vi "1.0-Hindbrain Global.vi"() -> ()   [LabVIEW 2010]
uses:
  2-Low Neurons/2.0-Hindbrain Startup State.ctl
  2-Low Neurons/2.1-Act Command Typedef.ctl
  2-Low Neurons/2.1 PID Gains Typedef.ctl
  2-Low Neurons/2.3-What Sensor Typedef.ctl
  2-Low Neurons/Data Latch.ctl
  2-Low Neurons/2.4-How Sensor Typedef.ctl
  2-Low Neurons/2.3.6-Decode State.ctl
  2-Low Neurons/2.7-Sense Queries Typedef.ctl
panel:
  out "Stop Loops":bool
  in  "Tab, for convenience":T1(tab)
  in  "2.1.3 Lidar Error D":fxp<+/-,18,1>
  in  "2.1.3 Lidar Error I":fxp<+/-,64,46>
  in  "2.1.3 Lidar Error":fxp<+/-,18,1>
  in  "2.1.2 Steering Error D":fxp<+/-,18,1>
  in  "2.1.2 Steering Error I":fxp<+/-,64,46>
  in  "2.1.2 Steering Error":fxp<+/-,18,1>
  in  "2.1.1 Drive Error D":fxp<+/-,18,1>
  in  "2.1.1 Drive Error I":fxp<+/-,64,46>
  in  "2.1.1 Drive Error":fxp<+/-,18,1>
  in  "2.1  Drive PID Output":fxp<+/-,20,5>
  in  "2.1  Lidar PID Output":fxp<+/-,20,5>
  in  "2.1  Steering PID Output":fxp<+/-,20,5>
  in  "2.1  Lidar Control Voltage":fxp<+/-,20,5>
  in  "2.1  Steering Control Voltage":fxp<+/-,20,5>
  in  "2.1 Drive Control Voltage":fxp<+/-,20,5>
  in  "2.1 Act Command":T2={"Inhibit All Motors"=FALSE, "2.1 Direct Override"=FALSE, "Drive Speed Integer Setpoint"=0, "Steering Integer Setpoint"=0, "Lidar Position Integer Setpoint"=0, "Drive Direct"=0.0, "Steer Direct"=0.0, "Lidar Direct "=0.0, "2.1.3 Drive PID Gains"={"P Gain"=0.25, "I Gain"=0.25, "D Gain"=0.25, "P Gain - Exp"=2, "I Gain - Exp"=2, "D Gain - Exp"=2}, "2.1.3 Steering PID Gains"={"P Gain"=0.25, "I Gain"=0.25, "D Gain"=0.25, "P Gain - Exp"=2, "I Gain - Exp"=2, "D Gain - Exp"=2}, "2.1.3 Lidar PID Gains"={"P Gain"=0.25, "I Gain"=0.25, "D Gain"=0.25, "P Gain - Exp"=2, "I Gain - Exp"=2, "D Gain - Exp"=2}, "2.5.5 A"=0.0, "2.5.6 B"=0.0, "Drive Limit"=0.0} {"2.1.3 Lidar PID Gains"."P Gain" format="%.8f"; "2.1.3 Lidar PID Gains"."I Gain" format="%.8f"; "2.1.3 Lidar PID Gains"."D Gain" format="%.8f"; "2.1.3 Drive PID Gains"."P Gain" format="%.8f"; "2.1.3 Drive PID Gains"."I Gain" format="%.8f"; "2.1.3 Drive PID Gains"."D Gain" format="%.8f"; "2.1.3 Steering PID Gains"."P Gain" format="%.8f"; "2.1.3 Steering PID Gains"."I Gain" format="%.8f"; "2.1.3 Steering PID Gains"."D Gain" format="%.8f"}
  out "2.2.4-VectorNav Query":bool
  out "2.2.4 Read TimedOut?":bool
  out "2.2.3 Write TimedOut?":bool
  out "2.2.2 VectorNav ReceivedByte":u8
  in  "2.2.2 VectorNav SendByte":u8
  in  "2.2.1 VectorNavCommand":u8[](array[numeric])=[36, 86, 78, 82, 82, 71, 44, 48, 46, 52, 55, 66]
  in  "2.2.1Send":bool
  in  "2.2.1 VectorNav Yaw":i16
  in  "2.2 Where am I? Sensor":T4
  in  "2.3 What is Around Me? Sensor":T5={"FPGA Raw Datalatch"=enum."Idle", "Drivable Path Integers"=[0, 0, 0, 0, 0, 0, 0, 0, 0, 0, 0, 0, 0, 0, 0, 0]}
  out "2.3.6-Decode State":T7
  out "2.3.3-Scan":u8
  out "2.3.7-Paths":u16[](array[numeric])
  out "2.3.4-X":i16
  out "2.3.5-Y":i16
  out "2.3.8-DMA Timeout":bool
  in  "2.4.5 FPGA LED Heart Beat Duty":u8
  in  "2.4.2.3 Reverse?":bool
  in  "2.4.4.2 Lidar V":fxp<+/-,10,8>
  in  "2.4.3.2 Lidar Mot V":fxp<+/-,10,8>
  in  "2.4.1.2 Steer V":fxp<+/-,10,8>
  in  "2.4.2.2 Drive V":fxp<+/-,10,8>
  in  "2.4.4.1 Lidar Pos":i32
  in  "2.4.3.1 Lidar Mot Pos":i32
  in  "2.4.2.1 Drive Pos":i32
  in  "2.4.1.1 Steer Pos":i32
  in  "2.4 How Am I? Sensor":T8
  in  "2.5.7 A*B":fxp<+/-,18,1>
  out "2.5.4-Timeouts by Identifier":bool[](array[boolean])
  in  "2.5.1-Write Index":u32
  out "2.7 Sense Queries":T9
  in  "Enum":T10=enum."Running"
  # "2.5.2-MultServ Out"
  # "2.5.3-MultServ In"
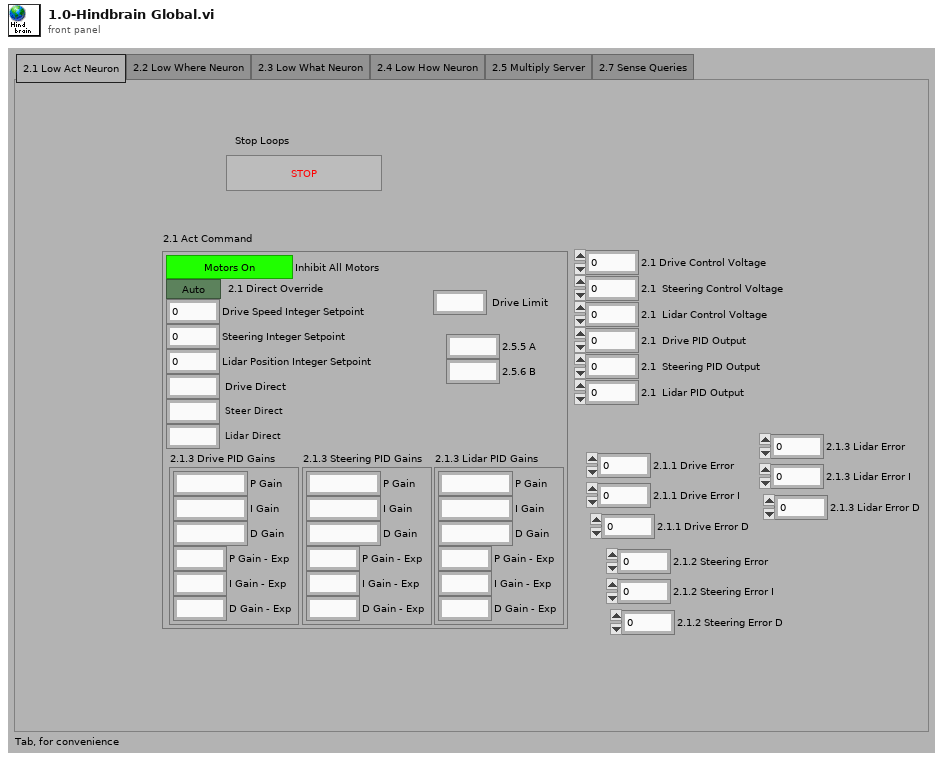
[diagram p1: front panel]
types:
  T1 = enum32{"2.1 Low Act Neuron", "2.2 Low Where Neuron", "2.3 Low What Neuron", "2.4 Low How Neuron", "2.5 Multiply Server", "2.7 Sense Queries"}
  T2 = typedef "2.1-Act Command Typedef.ctl" = cluster{"Inhibit All Motors":bool, "2.1 Direct Override":bool, "Drive Speed Integer Setpoint":i32, "Steering Integer Setpoint":i32, "Lidar Position Integer Setpoint":i32, "Drive Direct":fxp<+/-,20,5>, "Steer Direct":fxp<+/-,20,5>, "Lidar Direct ":fxp<+/-,20,5>, "2.1.3 Drive PID Gains":T3, "2.1.3 Steering PID Gains":T3, "2.1.3 Lidar PID Gains":T3, "2.5.5 A":fxp<+/-,18,1>, "2.5.6 B":fxp<+/-,18,1>, "Drive Limit":fxp<+/-,20,5>}
  T3 = typedef "2.1 PID Gains Typedef.ctl" = cluster{"P Gain":fxp<+/-,18,1>, "I Gain":fxp<+/-,18,1>, "D Gain":fxp<+/-,18,1>, "P Gain - Exp":i8, "I Gain - Exp":i8, "D Gain - Exp":i8}
  T4 = cluster{"INS X":i16, "INS Y":i16, "INS Z":i16, "INS Yaw":i16, "INS Raw":i8}
  T5 = typedef "2.3-What Sensor Typedef.ctl" = cluster{"FPGA Raw Datalatch":T6, "Drivable Path Integers":u16[]}
  T6 = typedef "Data Latch.ctl" = enum8{"Idle", "Sending", "Sent", "Receiving", "Received"}
  T7 = typedef "2.3.6-Decode State.ctl" = enum16{"wait for message start '['", "wait for point start '(' ", "record x value", "record y value", "scan complete"}
  T8 = typedef "2.4-How Sensor Typedef.ctl" = cluster{"Motor Speed Integer":i32, "Drive Position Integer":i32, "Lidar Position Integer":i32, "Lidar Motor Position Integer":i32, "Steering Position Integer":i32, "Battery Voltage Fxp":fxp<+/-,16,5>, "Drive Encoder Cable Check":bool, "Lidar Drive Encoder Cable Check":bool, "Steer Encoder Cable Check":bool, "Lidar Pos Encoder Cable Check":bool, "Mod Buttons & Blinky Cable Check":bool, "Lidar Data Cable Check":bool, "Drive Motor Cable Check":bool, "Vector Nav Cable Check":bool, "Lidar Drive Cable Check":bool, "Steer Drive Cable Check":bool, "Reverse?":bool, "2.1  Steering Control Voltage":fxp<+/-,20,5>, "2.1 Drive Control Voltage":fxp<+/-,20,5>, "2.1  Lidar Control Voltage":fxp<+/-,20,5>, "2.5.7 A*B":fxp<+/-,18,1>, "2.1  Steering PID Output":fxp<+/-,20,5>, "2.1 Drive PID Output":fxp<+/-,20,5>, "2.1  Lidar PID Output":fxp<+/-,20,5>, "2.1.1 Drive Error":fxp<+/-,18,1>, "2.1.1 Drive Error I":fxp<+/-,64,46>, "2.1.1 Drive Error D":fxp<+/-,18,1>, "2.1.2 Steering Error":fxp<+/-,18,1>, "2.1.2 Steering Error I":fxp<+/-,64,46>, "2.1.2 Steering Error D":fxp<+/-,18,1>, "2.1.3 Lidar Error":fxp<+/-,18,1>, "2.1.3 Lidar Error I":fxp<+/-,64,46>, "2.1.3 Lidar Error D":fxp<+/-,18,1>, "VectorNav Ack Query":bool}
  T9 = typedef "2.7-Sense Queries Typedef.ctl" = cluster{"VectorNav Query":bool}
  T10 = typedef "2.0-Hindbrain Startup State.ctl" = enum8{"Waiting to Run", "Running", "Restart", "Shutdown", "Off"}
diagram:
